vi "读取固件状态.vi"(8 "错误输入":errorcluster, 11 "MB session in":refnum<class "MB_Master.lvclass">) -> (0 "error out":errorcluster, 2 "结果字符串":string, 3 "MB session out":refnum<class "MB_Master.lvclass">)   [LabVIEW 2016, in "斯坦道总磷总氮.lvlib"]
uses:
  <vilib>/Plasmionique/MB Master/MB_Master/MB_Master.lvclass
  <vilib>/Plasmionique/MB Master/MB_Master_Serial/MB_Master_Serial.lvclass
  C:/Program Files (x86)/National Instruments/LabVIEW 2016/vi.lib/Plasmionique/MB Master/MB_Master/MB_Master.lvclass
  <vilib>/Plasmionique/MB Master/MB Master.lvlib
panel:
  in  "VISA Resource":refnum<visa-resource-name>
  in  "引用选择":enum16{"MB引用", "自建引用"}(ring)
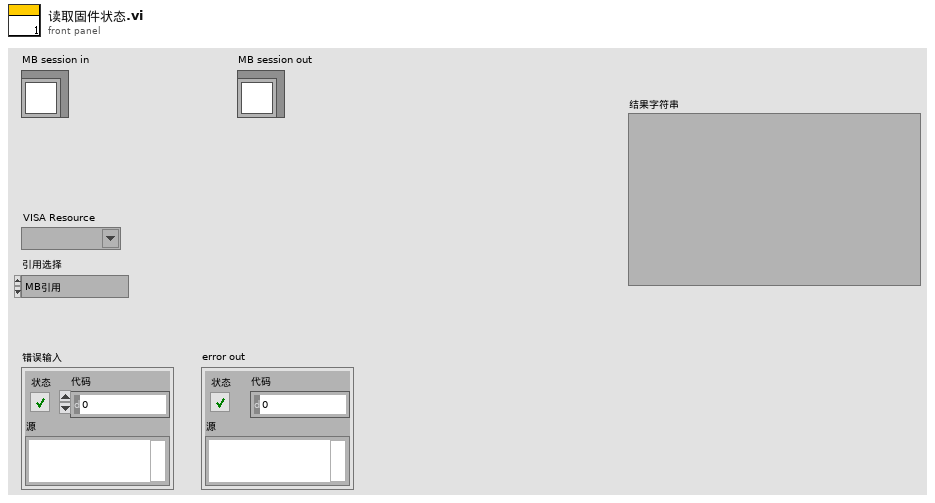
[diagram p1: front panel]
types:
  T1 = cluster{"baud rate (bps)":u32, "stop bits":u16, "parity":u16, "flow control":u16, "timeout":u32, "retries":i32}
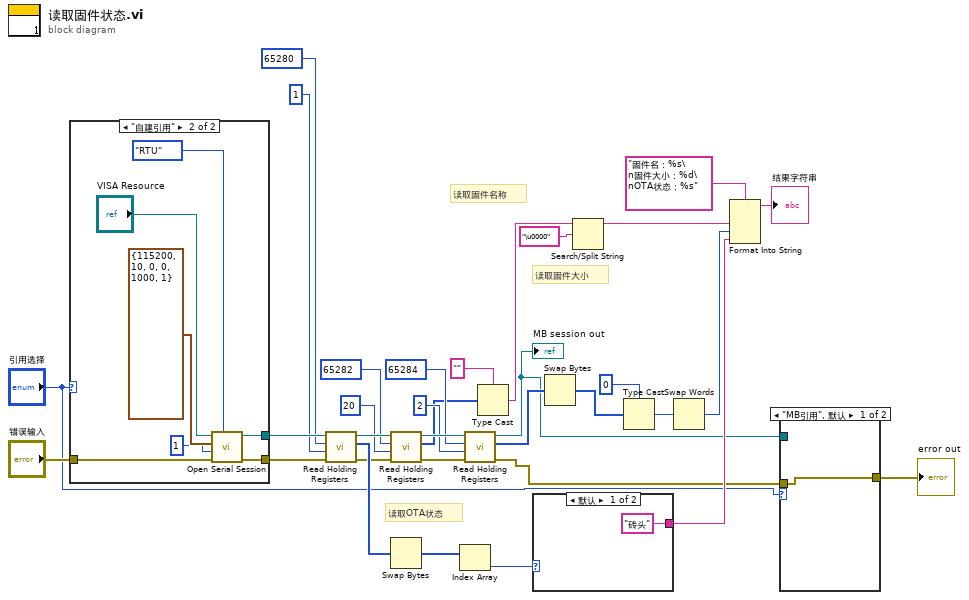
[diagram p0: block diagram]
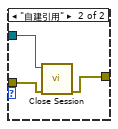
[diagram p2: hidden frame]
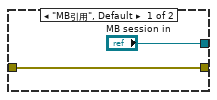
[diagram p3: hidden frame]
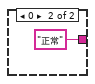
[diagram p4: hidden frame]
diagram:
  # "读取固件大小"
  # "读取固件名称"
  # "读取OTA状态"
  n1 = case shown="\"自建引用\"" "引用选择" {
    tunnel: ["MB session in" w41] -> w32
    tunnel: "错误输入" -> [w34 w40]
    tunnel: [w34 w39] -> w11
    frame "MB引用", Default {
    }
    frame "自建引用" {
      n2 = call <vilib>:"Open Serial Session.vi"("Mode (RTU)"=enum16{"RTU", "ASCII"}."RTU", "Error in"=w40, "Slave ID"=u8 1, "Serial Config"=T1 {"baud rate (bps)"=115200, "stop bits"=10, "parity"=0, "flow control"=0, "timeout"=1000, "retries"=1}, "VISA Resource"="VISA Resource") -> ("Error out"=w39:errorcluster, "MB_Serial session"=w41:refnum<class "MB_Master_Serial.lvclass">)  [unwired: 5 in]
    }
  }
  n3 = call <vilib>:"Read Holding Registers.vi"("error in (no error)"=w11, "quantity"=u16 1, "starting address"=u16 65280, "MB session in"=w32) -> ("error out"=w19:errorcluster, "Registers"=w29:u16[], "MB session out"=w24:refnum<class "MB_Master.lvclass">)  [unwired: 5 in]
  n4 = call <vilib>:"Read Holding Registers.vi"("error in (no error)"=w19, "quantity"=u16 20, "starting address"=u16 65282, "MB session in"=w24) -> ("error out"=w18:errorcluster, "Registers"=w5:u16[], "MB session out"=w22:refnum<class "MB_Master.lvclass">)  [unwired: 5 in]
  n5 = Swap Bytes(anything=w29) -> (byte swapped=w27:u16[])
  n6 = Index Array(array=w27) -> (element=w28:u16)  [unwired: 1 in]
  n7 = call <vilib>:"Read Holding Registers.vi"("error in (no error)"=w18, "quantity"=u16 2, "starting address"=u16 65284, "MB session in"=w22) -> ("error out"=w3:errorcluster, "Registers"=w17:u16[], "MB session out"=w4:refnum<class "MB_Master.lvclass">)  [unwired: 5 in]
  "MB session out" <- w4
  n8 = Type Cast(type="", x=w5) -> (*(type *) &x=w6:string)
  n9 = case shown="默认" w28 {
    tunnel: ["砖头" "正常"] -> w26
    frame Default {
    }
    frame 0 {
    }
  }
  n10 = Swap Bytes(anything=w17) -> (byte swapped=w16:u16[])
  n11 = Search/Split String(string=w6, search string/char (-)="\u0000" ("搜索字符串")) -> (substring before match=w8:string)  [unwired: 1 in, 2 out]
  n12 = Type Cast(type=u32 0, x=w16) -> (*(type *) &x=w14:u32)
  n13 = Swap Words(1:w14) -> (0:w13:u32)
  n14 = Format Into String(format string="固件名：%s\n固件大小：%d\nOTA状态：%s" ("格式字符串"), w8, w13, w26) -> (resulting string=→"结果字符串":string)  [unwired: 2 in, 1 out]
  n15 = case shown="\"MB引用\", 默认" "引用选择" {
    tunnel: w4 -> [_ w48]
    tunnel: w3 -> [w45 w47]
    tunnel: [w45 w46] -> w2
    frame "MB引用", Default {
    }
    frame "自建引用" {
      n16 = call-dynamic "Close Session.vi"("error in (no error)"=w47, "MB session in"=w48) -> ("error out"=w46:errorcluster)  [unwired: 9 in]
    }
  }
  "error out" <- w2
